vi "Read Array Key (DBL).vi"(7 "Section Name":string, 8 "error in (no error)":errorcluster, 9 "Default":dbl, 10 "Key Name":string, 11 "Config in":refnum<class "LabVIEW-Config.lvclass">) -> (0 "error out":errorcluster, 1 "Value":dbl[](array[numeric]), 2 "Key Found?":bool, 3 "Config out":refnum<class "LabVIEW-Config.lvclass">)   [LabVIEW 2017, in "LabVIEW-Config.lvlib" / "LabVIEW-Config.lvclass"]
uses:
  LabVIEW-Config.lvclass
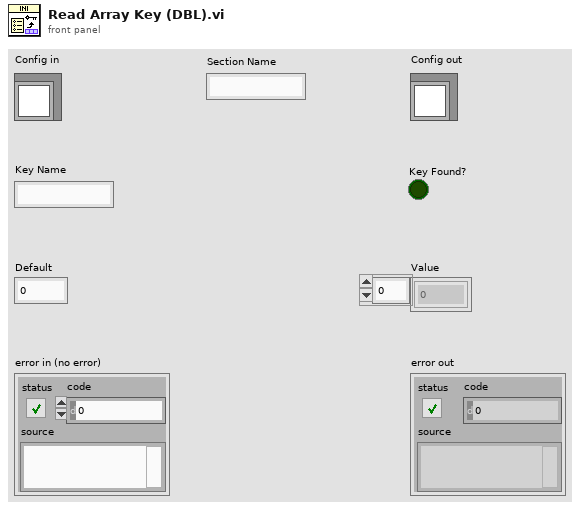
[diagram p1: front panel]
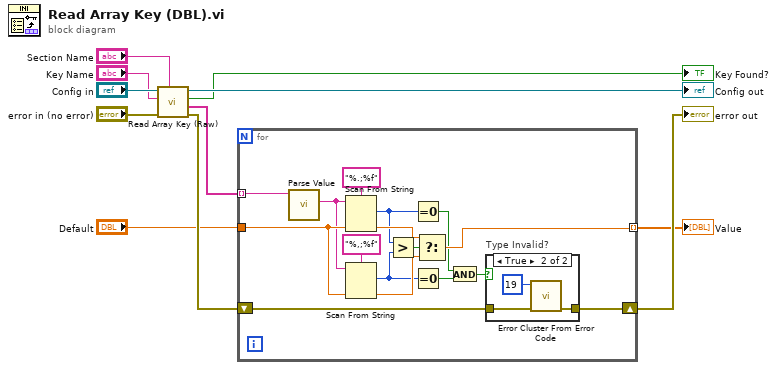
[diagram p0: block diagram]
diagram:
  n1 = call "Read Array Key (Raw).vi"("Section Name"="Section Name", "error in (no error)"="error in (no error)", "Key Name"="Key Name", "Config in"="Config in") -> ("error out"=w4:errorcluster, "Content"=w6:string[], "Key Found?"=→"Key Found?":bool, "Config out"=→"Config out":refnum<class "LabVIEW-Config.lvclass">)  [unwired: 4 in]
  n2 = for {
    tunnel: w6 -> [w27] mode=indexing
    shift-right: [w26] -> w5
    shift-left: w4 -> [w25]
    tunnel: "Default" -> [w24]
    tunnel: [w23] -> w1 mode=indexing
    n3 = call "Parse Value.vi"("Value"=w27) -> ("Value (Comment Removed)"=w13:string)  [unwired: 9 in, 1 out]
    n4 = Scan From String(format string="%.;%f" ("Format String"), input string=w13, default 1=w24) -> (offset past scan=w17:u32, output 1=w19:dbl)  [unwired: 2 in, 2 out]
    n5 = Scan From String(format string="%,;%f" ("Format String"), input string=w13, default 1=w24) -> (offset past scan=w16:u32, output 1=w18:dbl)  [unwired: 2 in, 2 out]
    n6 = Greater?(x=w17, y=w16) -> (0:w20:bool)
    n7 = Equal To 0?(x=w17) -> (x = 0?=w14:bool)
    n8 = Equal To 0?(x=w16) -> (x = 0?=w15:bool)
    n9 = Select(t=w19, s=w20, f=w18) -> (s? t:f=w23:dbl)
    n10 = And(x=w14, y=w15) -> (x .and. y?=w12:bool)
    n11 = case "Type Invalid?" shown="True" w12 {
      tunnel: w25 -> [w28 w30]
      tunnel: [w28 w29] -> w26
      frame False {
      }
      frame True {
        n12 = call <vilib>:"Error Cluster From Error Code.vi"("error in (no error)"=w30, "error code (0)"=19 ("Type invalid")) -> ("error out"=w29:errorcluster)  [unwired: 7 in]
      }
    }
  }
  "error out" <- w5
  "Value" <- w1
